vi "GetRobotPos.vi"(0 "Left Encoder":T1={"DevStatus"={"status"=FALSE, "code"=0, "source"=""}, "EncoderIndex"=enum."Invalid", "CounterIndex"=enum."Invalid", "DistancePerCount"=1.0, "Decoding Type"=enum."4x"}, 1 "Left Encoder In":dbl, 2 "X/Y/a In":T5, 3 "Right Encoder":T1={"DevStatus"={"status"=FALSE, "code"=0, "source"=""}, "EncoderIndex"=enum."Invalid", "CounterIndex"=enum."Invalid", "DistancePerCount"=1.0, "Decoding Type"=enum."4x"}, 4 "Right Encoder In":dbl) -> (5 "Left Encoder Out":dbl, 6 "X/Y/a Out":T5, 7 "Right Encoder Out":dbl)   [LabVIEW 2014]
uses:
  <vilib>/Rock Robotics/WPI/Encoder/WPI_EncoderDevRef.ctl
  <vilib>/Rock Robotics/SystemInterfaces/Encoder/FPGA_EncoderIdx.ctl
  <vilib>/Rock Robotics/SystemInterfaces/Counter/FPGA_CounterCtrSystemIndex.ctl
  <vilib>/Rock Robotics/WPI/Encoder/WPI_EncoderType.ctl
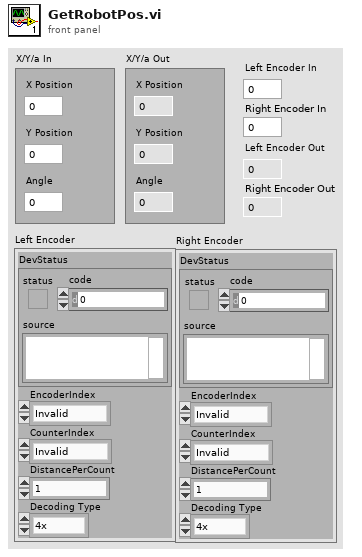
[diagram p1: front panel]
types:
  T1 = typedef "WPI_EncoderDevRef.ctl" = cluster{"DevStatus":errorcluster, "EncoderIndex":T2, "CounterIndex":T3, "DistancePerCount":dbl, "Decoding Type":T4}
  T2 = typedef "FPGA_EncoderIdx.ctl" = enum8{"Enc 0", "Enc 1", "Enc 2", "Enc 3", "Enc 4", "Enc 5", "Enc 6", "Enc 7", "Invalid"}
  T3 = typedef "FPGA_CounterCtrSystemIndex.ctl" = enum8{"Ctr 0", "Ctr 1", "Ctr 2", "Ctr 3", "Ctr 4", "Ctr 5", "Ctr 6", "Ctr 7", "Invalid"}
  T4 = typedef "WPI_EncoderType.ctl" = enum16{"1x", "2x", "4x"}
  T5 = cluster{"X Position":dbl, "Y Position":dbl, "Angle":dbl}
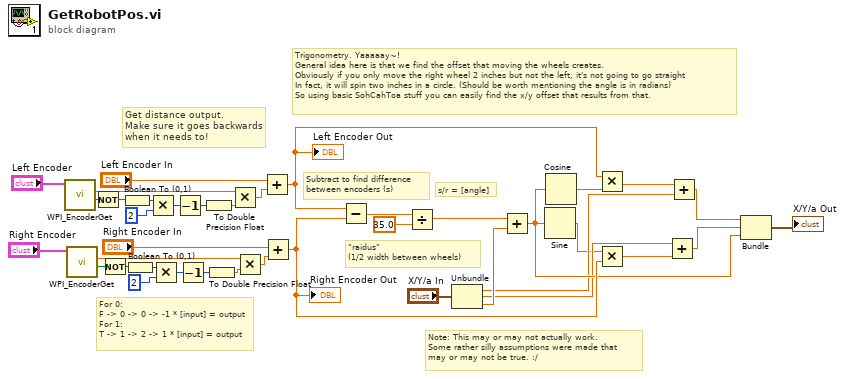
[diagram p0: block diagram]
diagram:
  # "For 0:\nF -> 0 -> 0 -> -1 * [input] = output\nFor 1:\nT -> 1 -> 2 -> 1 * [input] = output"
  # "Note: This may or may not actually work.\nSome rather silly assumptions were made that\nmay or may not be true. :/"
  # "\"raidus\" \n(1/2 width between wheels)"
  # "s/r = [angle]"
  # "Trigonometry. Yaaaaay~!\nGeneral idea here is that we find the offset that moving the wheels creates.\nObviously if you only move the right wheel 2 inches but not the left, it's not going to go straight\nIn fact, it will spin two inches in a circle. (Should be worth mentioning the angle is in radians)\nSo using basic SohCahToa stuff you can easily find the x/y offset that results from that."
  # "Get distance output.\nMake sure it goes backwards\nwhen it needs to!"
  # "Subtract to find difference\nbetween encoders (s)"
  n1 = call <vilib>:"WPI_EncoderGet.vi"("EncoderDevRef"="Left Encoder") -> ("Direction"=w17:bool, "Distance"=w36:dbl)  [unwired: 5 in, 4 out]
  n2 = call <vilib>:"WPI_EncoderGet.vi"("EncoderDevRef"="Right Encoder") -> ("Direction"=w26:bool, "Distance"=w34:dbl)  [unwired: 5 in, 4 out]
  n3 = Not(x=w17) -> (.not. x?=w15:bool)
  n4 = Not(x=w26) -> ()  [unwired: 1 out]
  n5 = Boolean To (0,1)(Boolean=w15) -> (0, 1=w20:i16)
  n6 = Boolean To (0,1)(Boolean=w26) -> (0, 1=w24:i16)
  n7 = Multiply(x=w20, y=i16 2) -> (x*y=w19:i16)
  n8 = Multiply(x=w24, y=i16 2) -> (x*y=w23:i16)
  n9 = Decrement(x=w19) -> (x-1=w18:i16)
  n10 = Decrement(x=w23) -> (x-1=w22:i16)
  n11 = To Double Precision Float(number=w18) -> (double precision float=w16:dbl)
  n12 = To Double Precision Float(number=w22) -> (double precision float=w35:dbl)
  n13 = Multiply(x=w36, y=w16) -> (x*y=w37:dbl)
  n14 = Multiply(x=w34, y=w35) -> (x*y=w32:dbl)
  n15 = Add(x="Left Encoder In", y=w37) -> (x+y=w28:dbl)
  "Left Encoder Out" <- w28
  n16 = Add(x="Right Encoder In", y=w32) -> (x+y=w27:dbl)
  "Right Encoder Out" <- w27
  n17 = Subtract(x=w28, y=w27) -> (x-y=w31:dbl)
  n18 = Divide(x=w31, y=35.0) -> (x/y=w29:dbl)
  n19 = Unbundle("X/Y/a In") -> ("X Position"=w3:dbl, "Y Position"=w2:dbl, "Angle"=w10:dbl)
  n20 = Add(x=w29, y=w10) -> (x+y=w6:dbl)
  n21 = Sine(x=w6) -> (sin(x)=w1:dbl)
  n22 = Cosine(x=w6) -> (cos(x)=w5:dbl)
  n23 = Multiply(x=w28, y=w5) -> (x*y=w4:dbl)
  n24 = Multiply(x=w1, y=w27) -> (x*y=w14:dbl)
  n25 = Add(x=w2, y=w14) -> (x+y=w7:dbl)
  n26 = Add(x=w4, y=w3) -> (x+y=w8:dbl)
  n27 = Bundle(w8, w7, w6) -> (→"X/Y/a Out":cluster{dbl, dbl, dbl})  [unwired: 1 in]
